vi "AIT 1553 - Write outgoing message data.vi"(4 "Bus Section":T1, 6 "Iteration":i32, 8 "error in (no error)":errorcluster, 9 "Msg Data In":u16[](array[numeric]), 10 "Values":dbl[](array[numeric]), 11 "Driver Data":T2 {"First Word" min=8 max=31; "Num Bits" min=1 max=32; "Start Bit" min=8 max=31}) -> (0 "error out":errorcluster, 1 "Msg Data Out":u16[](array[numeric]))   [LabVIEW 2013, in "AIT 1553 Custom Device.lvlib"]
uses:
  AIT 1553 Custom Device.lvlib
  RT Controls/AIT 1553 - Driver Data.ctl
  Controls and Global/Start Bit.ctl
  Controls and Global/Number of Bits.ctl
  RT Controls/AIT 1553 - Bus Section.ctl
  System Explorer/Controls/1553 Param.ctl
  <instrlib>/AIT 1553/AIT 1553.lvlib
  <vilib>/NI Veristand/Custom Device API/Global Data Refs.vi
  <vilib>/NI Veristand/Custom Device API/Custom Device API.lvlib
  <vilib>/NI Veristand/Custom Device Tools/Custom Device Utility Library/Custom Device Utility Library.lvlib
  <vilib>/NI Veristand/Custom Device Tools/Custom Device Utility Library/RT Debug String Color Spec.ctl
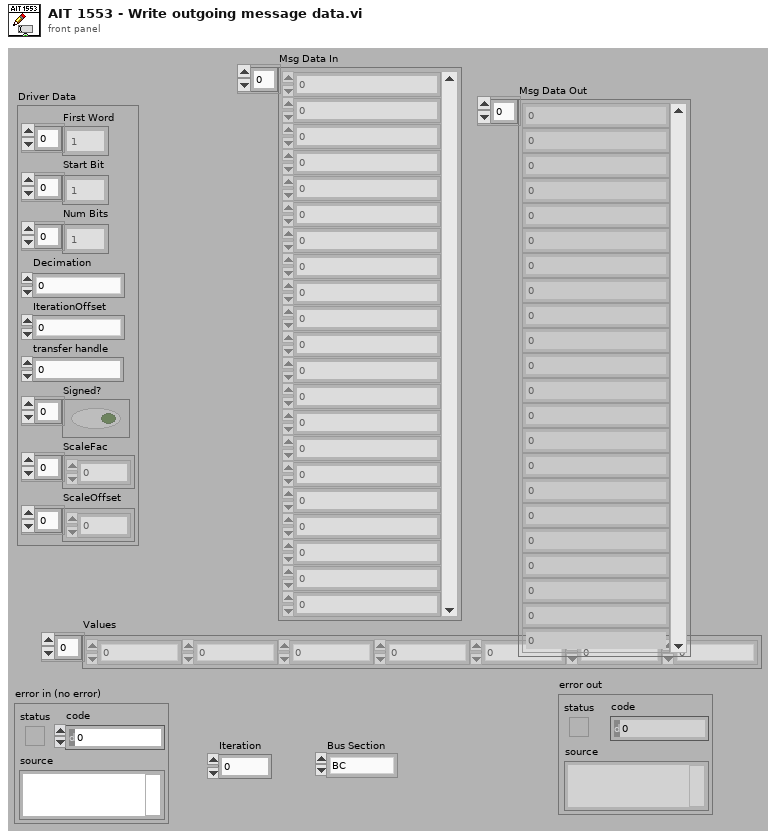
[diagram p1: front panel]
types:
  T1 = typedef "AIT 1553 Custom Device.lvlib/AIT 1553 - Bus Section.ctl" = enum16{"BC", "BM", "RT"}
  T2 = typedef "AIT 1553 Custom Device.lvlib/AIT 1553 - Driver Data.ctl" = cluster{"First Word":T3[], "Start Bit":T3[], "Num Bits":T4[], "Decimation":i32, "IterationOffset":i32, "transfer handle":u32, "Signed?":bool[], "ScaleFac":dbl[], "ScaleOffset":dbl[]}
  T3 = typedef "AIT 1553 Custom Device.lvlib/Start Bit.ctl" = i32
  T4 = typedef "AIT 1553 Custom Device.lvlib/Number of Bits.ctl" = i32
  T5 = typedef "AIT 1553 Custom Device.lvlib/1553 Param.ctl" = cluster{"name":string, "firstWord":i32, "startBit":i32, "numberBits":i32, "scaleFactor":dbl, "scaleOffset":dbl, "signed":bool}
  T6 = typedef "Custom Device Utility Library.lvlib/RT Debug String Color Spec.ctl" = u16
  T7 = typedef "Custom Device API.lvlib/Data Table Ref.ctl" = cluster{"Ptr.Beg":i32, "Ptr.End":i32}
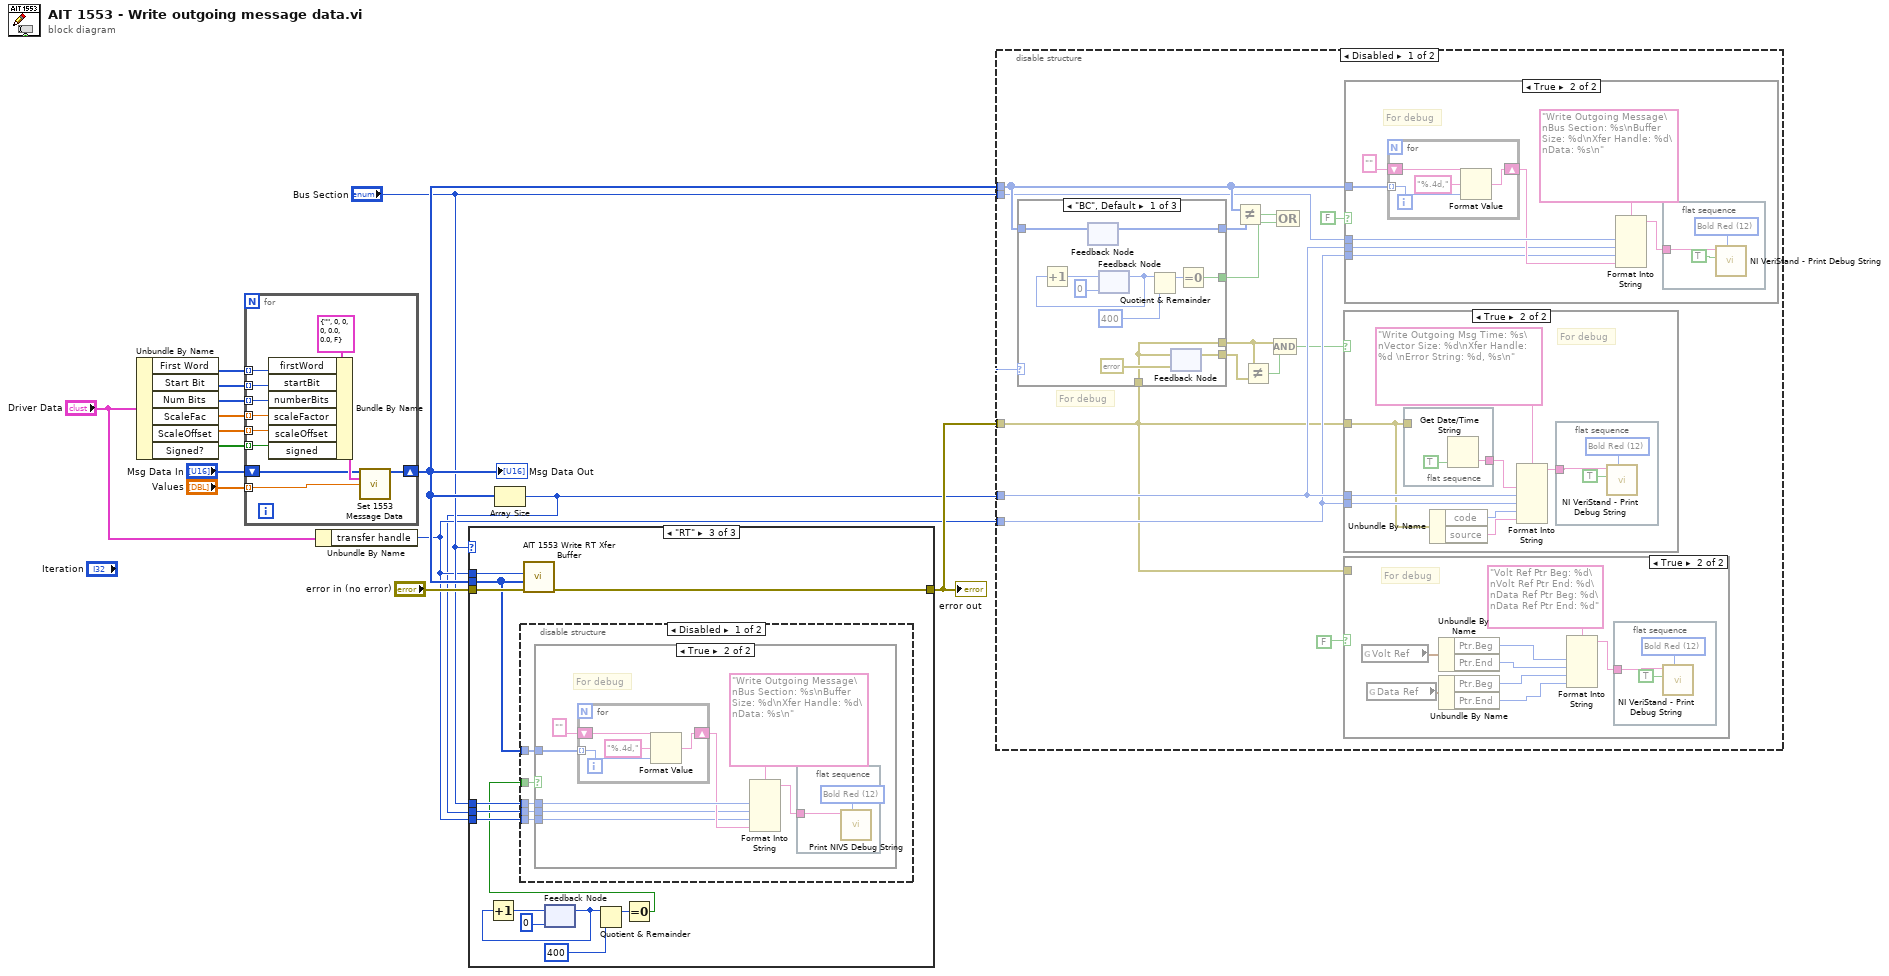
[diagram p0: block diagram]
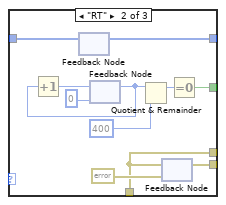
[diagram p2: hidden frame]
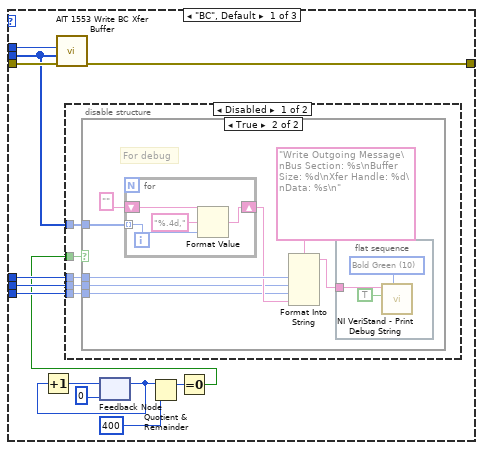
[diagram p8: hidden frame]
diagram:
  n1 = Unbundle By Name("Driver Data") -> ("First Word"=w15:T3[], "Start Bit"=w14:T3[], "Num Bits"=w13:T4[], "ScaleFac"=w12:dbl[], "ScaleOffset"=w11:dbl[], "Signed?"=w10:bool[])
  n2 = for {
    tunnel: w15 -> [w25] mode=indexing
    tunnel: w14 -> [w24] mode=indexing
    tunnel: w13 -> [w23] mode=indexing
    tunnel: w12 -> [w22] mode=indexing
    tunnel: w11 -> [w21] mode=indexing
    tunnel: w10 -> [w20] mode=indexing
    tunnel: "Values" -> [w17] mode=indexing
    shift-right: [w16] -> w6
    shift-left: "Msg Data In" -> [w18]
    n3 = Bundle By Name(cluster=T5 {"name"="", "firstWord"=0, "startBit"=0, "numberBits"=0, "scaleFactor"=0.0, "scaleOffset"=0.0, "signed"=FALSE} ("1553 Parameter"), "firstWord"=w25, "startBit"=w24, "numberBits"=w23, "scaleFactor"=w22, "scaleOffset"=w21, "signed"=w20) -> (w19:T5)
    n4 = call "Set 1553 Message Data.vi"("MSG DATA In"=w18, "1553 Parameter"=w19, "Value"=w17) -> ("MSG DATA Out"=w16:u16[])  [unwired: 11 in, 1 out]
  }
  "Msg Data Out" <- w6
  n5 = Unbundle By Name("Driver Data") -> ("transfer handle"=w2:u32)
  n6 = Array Size(array=w6) -> (size(s)=w1:i32)
  n7 = case shown="\"RT\"" "Bus Section" {
    tunnel: "error in (no error)" -> [w39 w60 w73]
    tunnel: w6 -> [w31 _ w70]
    tunnel: w2 -> [w38 _ w71]
    tunnel: [w37 w60 w72] -> w5
    tunnel: "Bus Section" -> [w30 _ w69]
    tunnel: w2 -> [w28 _ w68]
    tunnel: w1 -> [w29 _ w67]
    frame "BC", Default {
      n8 = call <instrlib>:"AIT 1553 Write BC Xfer Buffer.vi"("error in"=w39, "source buffer in"=w31, "BC transfer handle in"=w38) -> ("error out"=w37:errorcluster)  [unwired: 7 in, 1 out]
      n9 = feedback #1(0) -> (w32:i32)
      n10 = Increment(x=w32) -> (x+1=w34:i32)
      n11 = feedback-in #1(w34) -> ()
      n12 = Quotient & Remainder(x=w32, y=400) -> (x-y*floor(x/y)=w36:i32)  [unwired: 1 out]
      n13 = Equal To 0?(x=w36) -> (x = 0?=w27:bool)
      n14 = disable-structure shown="Disabled" {
        disable-tunnel: w31 -> [w44 _]
        disable-tunnel: w30 -> [w43 _]
        disable-tunnel: w29 -> [w42 _]
        disable-tunnel: w28 -> [w41 _]
        disable-tunnel: w27 -> [w40 _]
        frame Disabled {
          n15 = case shown="True" w40 {
            tunnel: w43 -> [_ w50]
            tunnel: w44 -> [_ w49]
            tunnel: w42 -> [_ w46]
            tunnel: w41 -> [_ w45]
            frame False {
            }
            frame True {
              # "For debug"
              n16 = for {
                tunnel: w49 -> [w53] mode=indexing
                shift-right: [w54] -> w47
                shift-left: "" ("format string") -> [w55]
                n17 = Format Value(string ("")=w55, format string="%.4d,", value (0)=w53) -> (output string=w54:string)
              }
              n18 = Format Into String(format string="Write Outgoing Message\nBus Section: %s\nBuffer Size: %d\nXfer Handle: %d\nData: %s\n", w50, w46, w45, w47) -> (resulting string=w51:string)  [unwired: 2 in, 1 out]
              n19 = flat-sequence {
                tunnel: w51 -> [w57]
                frame #0 {
                  w58 = T6 10 items=["Plain White"=7, "Bold White"=15, "Bold Blue"=9, "Bold Green"=10, "Bold Red"=12] ("Attribute")
                  n20 = call <vilib>:"NI VeriStand - Print Debug String.vi"("Attribute"=w58, "Add to log file? (T)"=TRUE, "Message"=w57) -> ()  [unwired: 8 in, 1 out]
                }
              }
            }
          }
        }
        frame Enabled {
        }
      }
    }
    frame "BM" {
    }
    frame "RT" {
      n21 = call <instrlib>:"AIT 1553 Write RT Xfer Buffer.vi"("error in"=w73, "source buffer in"=w70, "RT transfer handle in"=w71) -> ("error out"=w72:errorcluster)  [unwired: 7 in, 1 out]
      n22 = feedback #2(0) -> (w62:i32)
      n23 = Increment(x=w62) -> (x+1=w64:i32)
      n24 = feedback-in #2(w64) -> ()
      n25 = Quotient & Remainder(x=w62, y=400) -> (x-y*floor(x/y)=w66:i32)  [unwired: 1 out]
      n26 = Equal To 0?(x=w66) -> (x = 0?=w61:bool)
      n27 = disable-structure shown="Disabled" {
        disable-tunnel: w70 -> [w78 _]
        disable-tunnel: w69 -> [w77 _]
        disable-tunnel: w68 -> [w76 _]
        disable-tunnel: w67 -> [w75 _]
        disable-tunnel: w61 -> [w74 _]
        frame Disabled {
          n28 = case shown="True" w74 {
            tunnel: w77 -> [_ w84]
            tunnel: w78 -> [_ w83]
            tunnel: w75 -> [_ w80]
            tunnel: w76 -> [_ w79]
            frame False {
            }
            frame True {
              # "For debug"
              n29 = for {
                tunnel: w83 -> [w87] mode=indexing
                shift-right: [w88] -> w81
                shift-left: "" ("format string") -> [w89]
                n30 = Format Value(string ("")=w89, format string="%.4d,", value (0)=w87) -> (output string=w88:string)
              }
              n31 = Format Into String(format string="Write Outgoing Message\nBus Section: %s\nBuffer Size: %d\nXfer Handle: %d\nData: %s\n", w84, w80, w79, w81) -> (resulting string=w85:string)  [unwired: 2 in, 1 out]
              n32 = flat-sequence {
                tunnel: w85 -> [w91]
                frame #0 {
                  w92 = u16 12 items=["Plain White"=7, "Bold White"=15, "Bold Blue"=9, "Bold Green"=10, "Bold Red"=12] ("Color (Plain White)")
                  n33 = call "Print NIVS Debug String.vi"("Color (Plain White)"=w92, "Debug String"=w91) -> ()  [unwired: 8 in, 1 out]
                }
              }
            }
          }
        }
        frame Enabled {
        }
      }
    }
  }
  "error out" <- w5
  n34 = disable-structure shown="Disabled" {
    disable-tunnel: w1 -> [w106 _]
    disable-tunnel: w2 -> [w105 _]
    disable-tunnel: w6 -> [w102 _]
    disable-tunnel: "Bus Section" -> [w99 _]
    disable-tunnel: w5 -> [w93 _]
    frame Disabled {
      # "For debug"
      n35 = case shown="\"BC\", Default" w99 {
        tunnel: [w112 w123 _] -> w95
        tunnel: w102 -> [w111 w122 w129]
        tunnel: [w110 w121 w129] -> w101
        tunnel: w93 -> [w108 w119 _]
        tunnel: [w108 w119 _] -> w97
        tunnel: [w107 w118 _] -> w98
        frame "BC", Default {
          n36 = feedback #3() -> (w110:u16[])  [unwired: 1 in]
          n37 = feedback-in #3(w111) -> ()
          n38 = feedback #4(0) -> (w113:i32)
          n39 = Increment(x=w113) -> (x+1=w115:i32)
          n40 = feedback-in #4(w115) -> ()
          n41 = Quotient & Remainder(x=w113, y=400) -> (x-y*floor(x/y)=w117:i32)  [unwired: 1 out]
          n42 = feedback #5(errorcluster {"status"=FALSE, "code"=0, "source"=""} ("error out")) -> (w107:errorcluster)
          n43 = feedback-in #5(w108) -> ()
          n44 = Equal To 0?(x=w117) -> (x = 0?=w112:bool)
        }
        frame "RT" {
          n45 = feedback #6() -> (w121:u16[])  [unwired: 1 in]
          n46 = feedback-in #6(w122) -> ()
          n47 = feedback #7(0) -> (w124:i32)
          n48 = Increment(x=w124) -> (x+1=w126:i32)
          n49 = feedback-in #7(w126) -> ()
          n50 = Quotient & Remainder(x=w124, y=400) -> (x-y*floor(x/y)=w128:i32)  [unwired: 1 out]
          n51 = feedback #8(errorcluster {"status"=FALSE, "code"=0, "source"=""} ("error out")) -> (w118:errorcluster)
          n52 = feedback-in #8(w119) -> ()
          n53 = Equal To 0?(x=w128) -> (x = 0?=w123:bool)
        }
        frame "BM" {
        }
      }
      n54 = Not Equal?(x=w102, y=w101) -> (x != y?=w100:bool)
      n55 = Not Equal?(x=w97, y=w98) -> (x != y?=w104:bool)
      n56 = Compound Arithmetic op=AND(w97, w104) -> (w103:bool)
      n57 = Compound Arithmetic op=OR(w100, w95) -> ()  [unwired: 1 out]
      n58 = case shown="True" w103 {
        tunnel: w106 -> [_ w160]
        tunnel: w105 -> [_ w158]
        tunnel: w93 -> [_ w156]
        frame False {
        }
        frame True {
          # "For debug"
          n59 = flat-sequence {
            tunnel: [w165] -> w161
            tunnel: w156 -> [_]
            frame #0 {
              n60 = Get Date/Time String(want seconds? (F)=TRUE) -> (time string=w165:string)  [unwired: 2 in, 1 out]
            }
          }
          n61 = Unbundle By Name(w156) -> ("code"=w157:i32, "source"=w159:string)
          n62 = Format Into String(format string="Write Outgoing Msg Time: %s\nVector Size: %d\nXfer Handle: %d \nError String: %d, %s\n", w161, w160, w158, w157, w159) -> (resulting string=w163:string)  [unwired: 2 in, 1 out]
          n63 = flat-sequence {
            tunnel: w163 -> [w166]
            frame #0 {
              w167 = T6 12 items=["Plain White"=7, "Bold White"=15, "Bold Blue"=9, "Bold Green"=10, "Bold Red"=12] ("Attribute")
              n64 = call <vilib>:"NI VeriStand - Print Debug String.vi"("Attribute"=w167, "Add to log file? (T)"=TRUE, "Message"=w166) -> ()  [unwired: 8 in, 1 out]
            }
          }
        }
      }
      n65 = case shown="True" FALSE {
        tunnel: w93 -> [_ _]
        frame False {
        }
        frame True {
          # "For debug"
          n66 = global read "Global Data Refs.vi" "Volt Ref"() -> (w150:T7)
          n67 = global read "Global Data Refs.vi" "Data Ref"() -> (w149:T7)
          n68 = Unbundle By Name(w150) -> ("Ptr.Beg"=w148:i32, "Ptr.End"=w145:i32)
          n69 = Unbundle By Name(w149) -> ("Ptr.Beg"=w146:i32, "Ptr.End"=w147:i32)
          n70 = Format Into String(format string="Volt Ref Ptr Beg: %d\nVolt Ref Ptr End: %d\nData Ref Ptr Beg: %d\nData Ref Ptr End: %d", w148, w145, w146, w147) -> (resulting string=w151:string)  [unwired: 2 in, 1 out]
          n71 = flat-sequence {
            tunnel: w151 -> [w153]
            frame #0 {
              w154 = T6 12 items=["Plain White"=7, "Bold White"=15, "Bold Blue"=9, "Bold Green"=10, "Bold Red"=12] ("Attribute")
              n72 = call <vilib>:"NI VeriStand - Print Debug String.vi"("Attribute"=w154, "Add to log file? (T)"=TRUE, "Message"=w153) -> ()  [unwired: 8 in, 1 out]
            }
          }
        }
      }
      n73 = case shown="True" FALSE {
        tunnel: w99 -> [_ w135]
        tunnel: w102 -> [_ w134]
        tunnel: w106 -> [_ w131]
        tunnel: w105 -> [_ w130]
        frame False {
        }
        frame True {
          # "For debug"
          n74 = for {
            tunnel: w134 -> [w138] mode=indexing
            shift-right: [w139] -> w132
            shift-left: "" ("format string") -> [w140]
            n75 = Format Value(string ("")=w140, format string="%.4d,", value (0)=w138) -> (output string=w139:string)
          }
          n76 = Format Into String(format string="Write Outgoing Message\nBus Section: %s\nBuffer Size: %d\nXfer Handle: %d\nData: %s\n", w135, w131, w130, w132) -> (resulting string=w136:string)  [unwired: 2 in, 1 out]
          n77 = flat-sequence {
            tunnel: w136 -> [w142]
            frame #0 {
              w143 = T6 12 items=["Plain White"=7, "Bold White"=15, "Bold Blue"=9, "Bold Green"=10, "Bold Red"=12] ("Attribute")
              n78 = call <vilib>:"NI VeriStand - Print Debug String.vi"("Attribute"=w143, "Add to log file? (T)"=TRUE, "Message"=w142) -> ()  [unwired: 8 in, 1 out]
            }
          }
        }
      }
    }
    frame Enabled {
    }
  }
